vi "Create.vi"(10 "VolatusAPI":refnum<class "VolatusAPI.lvclass">) -> (3 "VolatusApiHttpService out":refnum<class "VolatusApiHttpService.lvclass">)   [LabVIEW 2020, in "Volatus.lvlib" / "VolatusApiHttpService.lvclass"]
uses:
  VolatusApiHttpService.lvclass
  VolatusApiHttpService.lvclass/VolatusApiHttpService.ctl
  VolatusAPI/VolatusAPI.lvclass
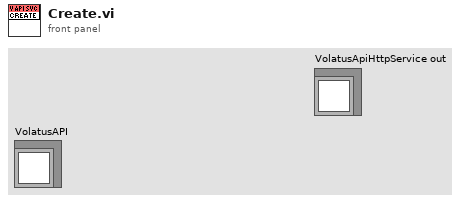
[diagram p1: front panel]
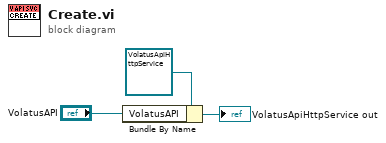
[diagram p0: block diagram]
diagram:
  n1 = Bundle By Name(cluster=refnum<class "VolatusApiHttpService.lvclass"> refnum ("VolatusApiHttpService out"), "VolatusAPI"="VolatusAPI") -> (→"VolatusApiHttpService out":refnum<class "VolatusApiHttpService.lvclass">)
